vi "Set_Init_States.vi"(4 "error in":errorcluster, 5 "register 2 (8-13)":T1=[FALSE, FALSE, FALSE, FALSE, FALSE, FALSE], 6 "register 1 (2-7)":T2=[FALSE, FALSE, FALSE, FALSE, FALSE, FALSE], 7 "Filename (ini)":string="Config_Ver_1\\pulse_sequence.ini") -> (0 "error out":errorcluster)   [LabVIEW 2021]
uses:
  Drivers/Arduino_Pulse_Generator/Configurate/Register_1.ctl
  Drivers/Arduino_Pulse_Generator/Configurate/Register_2.ctl
  <vilib>/Utility/config.llb/Write Key (Boolean).vi
  <vilib>/Utility/config.llb/NI_LVConfig.lvlib
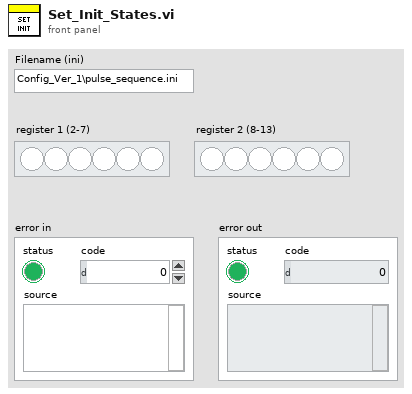
[diagram p1: front panel]
types:
  T1 = typedef "Register_2.ctl" = bool[]
  T2 = typedef "Register_1.ctl" = bool[]
  T3 = typedef "NI_LVConfig.lvlib/Config Data RefNum.ctl" = refnum<k1>
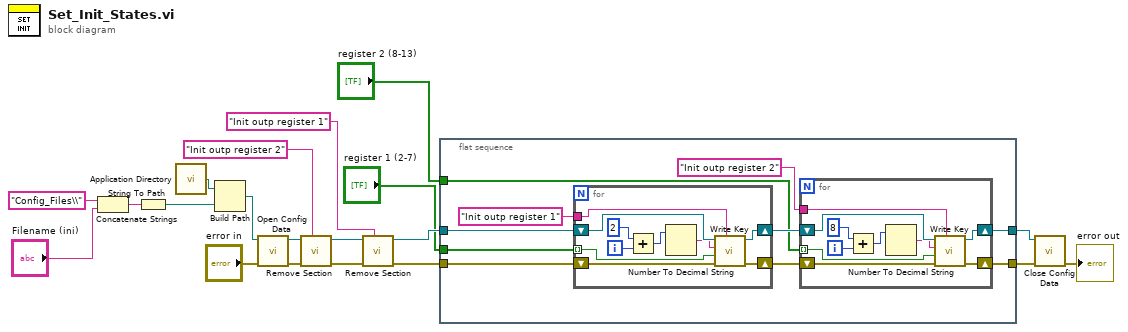
[diagram p0: block diagram]
diagram:
  n1 = Concatenate Strings("Config_Files\\" ("string"), "Filename (ini)") -> (w16:string)
  n2 = String To Path(string=w16) -> (path=w14:path)
  n3 = call <vilib>:"Application Directory.vi"() -> ("Application Directory"=w4:path)
  n4 = Build Path(base path=w4, name or relative path=w14) -> (appended path=w12:path)
  n5 = call <vilib>:"Open Config Data.vi"("error in (no error)"="error in", "configuration file path"=w12) -> ("error out"=w20:errorcluster, "refnum"=w19:T3)  [unwired: 7 in, 1 out]
  n6 = call <vilib>:"Remove Section.vi"("section"="Init outp register 2", "error in (no error)"=w20, "refnum"=w19) -> ("error out"=w17:errorcluster, "refnum out"=w18:T3)  [unwired: 6 in, 1 out]
  n7 = call <vilib>:"Remove Section.vi"("section"="Init outp register 1", "error in (no error)"=w17, "refnum"=w18) -> ("error out"=w3:errorcluster, "refnum out"=w11:T3)  [unwired: 6 in, 1 out]
  n8 = flat-sequence {
    tunnel: w3 -> [w30]
    tunnel: w11 -> [w29]
    tunnel: [w24] -> w8
    tunnel: [w23] -> w9
    tunnel: "register 2 (8-13)" -> [w22]
    tunnel: "register 1 (2-7)" -> [w21]
    frame #0 {
      n9 = for {
        tunnel: w21 -> [w44] mode=indexing
        shift-right: [w49] -> w27
        shift-left: w30 -> [w47]
        shift-right: [w48] -> w26
        shift-left: w29 -> [w50]
        tunnel: "Init outp register 1" ("section") -> [w41]
        i -> [w46]
        n10 = Add(x=2, y=w46) -> (x+y=w43:i32)
        n11 = Number To Decimal String(number=w43) -> (decimal integer string=w42:string)  [unwired: 1 in]
        n12 = call-poly <vilib>:"Write Key.vi"("section"=w41, "error in (no error)"=w47, "value"=w44, "key"=w42, "refnum"=w50) -> ("error out"=w49:errorcluster, "refnum out"=w48:T3)  [unwired: 4 in, 1 out]
      }
      n13 = for {
        tunnel: w22 -> [w34] mode=indexing
        shift-right: [w39] -> w24
        shift-left: w27 -> [w37]
        shift-right: [w38] -> w23
        shift-left: w26 -> [w40]
        tunnel: "Init outp register 2" ("section") -> [w31]
        i -> [w36]
        n14 = Add(x=8, y=w36) -> (x+y=w33:i32)
        n15 = Number To Decimal String(number=w33) -> (decimal integer string=w32:string)  [unwired: 1 in]
        n16 = call-poly <vilib>:"Write Key.vi"("section"=w31, "error in (no error)"=w37, "value"=w34, "key"=w32, "refnum"=w40) -> ("error out"=w39:errorcluster, "refnum out"=w38:T3)  [unwired: 4 in, 1 out]
      }
    }
  }
  n17 = call <vilib>:"Close Config Data.vi"("error in (no error)"=w8, "refnum"=w9) -> ("error out"=→"error out":errorcluster)  [unwired: 8 in, 1 out]
